vi "KMAX config write.vi"(0 "XScale.Maximum":dbl, 4 "XScale.Minimum":dbl, 6 "Integration Time (5 ms)":dbl=6000.0, 8 "Autoscale":bool, 9 "Camera Name":refnum<k21> caption="IMAQdx Session", 10 "Background":bool, 11 "configuration file path":path) -> ()   [LabVIEW 2023]
uses:
  <vilib>/Utility/config.llb/Write Key (Double).vi
  <vilib>/Utility/config.llb/Write Key (Boolean).vi
  <vilib>/Utility/config.llb/Write Key (String).vi
  <vilib>/Utility/config.llb/NI_LVConfig.lvlib
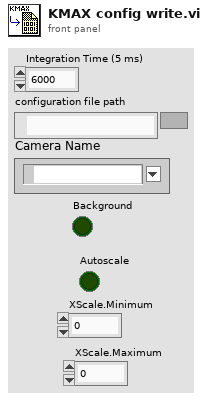
[diagram p1: front panel]
types:
  T1 = typedef "NI_LVConfig.lvlib/Config Data RefNum.ctl" = refnum<k1>
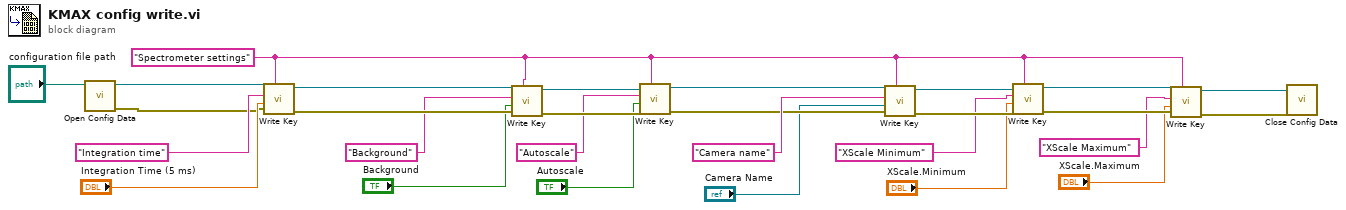
[diagram p0: block diagram]
diagram:
  w12 = "Spectrometer settings" ("section")
  n1 = call <vilib>:"Open Config Data.vi"("configuration file path"="configuration file path") -> ("error out"=w25:errorcluster, "refnum"=w28:T1)  [unwired: 8 in, 1 out]
  n2 = call-poly <vilib>:"Write Key.vi"("section"=w12, "error in (no error)"=w25, "value"="Integration Time (5 ms)", "key"="Integration time", "refnum"=w28) -> ("error out"=w8:errorcluster, "refnum out"=w11:T1)  [unwired: 4 in, 1 out]
  n3 = call-poly <vilib>:"Write Key.vi"("section"=w12, "error in (no error)"=w8, "value"="Background", "key"="Background", "refnum"=w11) -> ("error out"=w7:errorcluster, "refnum out"=w10:T1)  [unwired: 4 in, 1 out]
  n4 = call-poly <vilib>:"Write Key.vi"("section"=w12, "error in (no error)"=w7, "value"="Autoscale", "key"="Autoscale", "refnum"=w10) -> ("error out"=w6:errorcluster, "refnum out"=w9:T1)  [unwired: 4 in, 1 out]
  n5 = call-poly <vilib>:"Write Key.vi"("section"=w12, "error in (no error)"=w6, "value"="Camera Name", "key"="Camera name", "refnum"=w9) -> ("error out"=w22:errorcluster, "refnum out"=w19:T1)  [unwired: 4 in, 1 out]
  n6 = call-poly <vilib>:"Write Key.vi"("section"=w12, "error in (no error)"=w22, "value"="XScale.Minimum", "key"="XScale Minimum", "refnum"=w19) -> ("error out"=w21:errorcluster, "refnum out"=w18:T1)  [unwired: 4 in, 1 out]
  n7 = call-poly <vilib>:"Write Key.vi"("section"=w12, "error in (no error)"=w21, "value"="XScale.Maximum", "key"="XScale Maximum", "refnum"=w18) -> ("error out"=w20:errorcluster, "refnum out"=w17:T1)  [unwired: 4 in, 1 out]
  n8 = call <vilib>:"Close Config Data.vi"("error in (no error)"=w20, "refnum"=w17) -> ()  [unwired: 8 in, 2 out]
